vi "Read STATUS cluster.vi"(8 "error in (no error)":errorcluster, 11 "GSstatus in":refnum<class "GSstatus.lvclass">) -> (0 "error out":errorcluster, 2 "STATUS cluster":T1, 3 "GSstatus out":refnum<class "GSstatus.lvclass">)   [LabVIEW 2018, in "GSstatus.lvclass"]
uses:
  GSstatus.lvclass
  GSstatus.lvclass/GSstatus.ctl
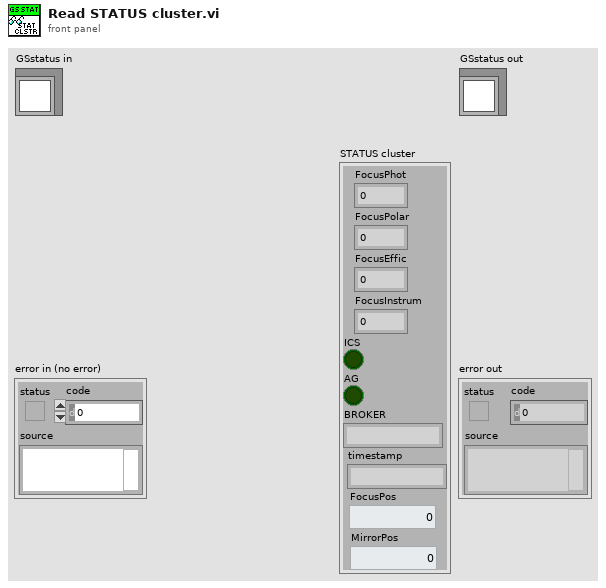
[diagram p1: front panel]
types:
  T1 = cluster{"FocusPhot":dbl, "FocusPolar":dbl, "FocusEffic":dbl, "FocusInstrum":dbl, "ICS":bool, "AG":bool, "BROKER":string, "timestamp":string, "FocusPos":dbl, "MirrorPos":dbl}
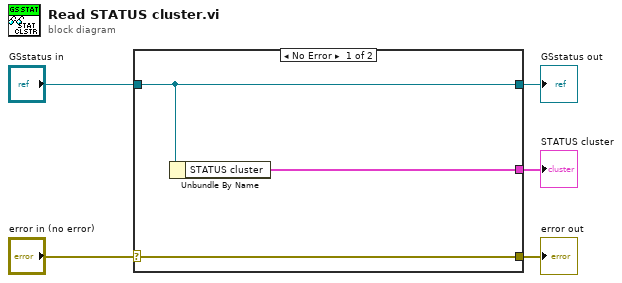
[diagram p0: block diagram]
diagram:
  n1 = case shown="No Error" "error in (no error)" {
    selector: "error in (no error)" -> [w8 w9]
    tunnel: [w8 w9] -> w4
    tunnel: [w7 w10] -> w2
    tunnel: "GSstatus in" -> [w7 w10]
    tunnel: [w6 _] -> w1
    frame No Error {
      n2 = Unbundle By Name(w7) -> ("STATUS cluster"=w6:T1)
    }
    frame Error {
    }
  }
  "error out" <- w4
  "GSstatus out" <- w2
  "STATUS cluster" <- w1
